vi "Read All Analog.vi"(0 "connection ID":refnum<k16>, 1 "address":u32, 2 "port":u16, 9 "timeout ms (1000)":i32=1000, 11 "error in (no error)":errorcluster) -> (4 "connection ID out":refnum<k16>, 6 "received data":string, 8 "Analog Values":u16[](array[numeric]), 15 "error out":errorcluster)   [LabVIEW 2016, in "instr.lvlib"]
doc: "Reads analog value all analog inputs and returns them as an array."
uses:
  instr.lvlib
panel:
  out "Send String":string
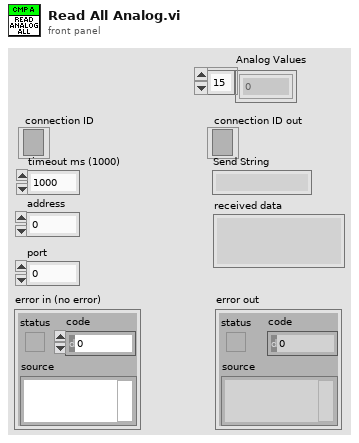
[diagram p1: front panel]
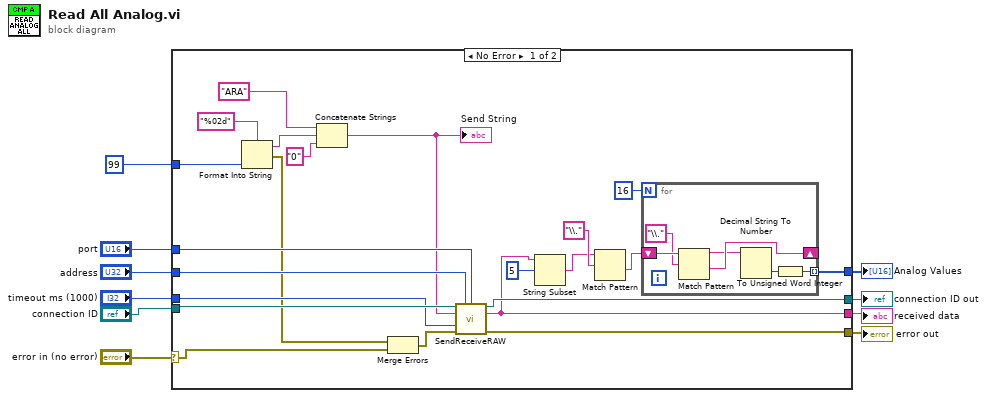
[diagram p0: block diagram]
diagram:
  n1 = case shown="No Error" "error in (no error)" {
    selector: "error in (no error)" -> [w22 w40]
    tunnel: [w32 w40] -> w10
    tunnel: "timeout ms (1000)" -> [w29 _]
    tunnel: "connection ID" -> [w30 w39]
    tunnel: [w31 w39] -> w6
    tunnel: "address" -> [w28 _]
    tunnel: "port" -> [w27 _]
    tunnel: [w12 _] -> w3
    tunnel: u16 99 ("Analog Number") -> [w23 _]
    tunnel: [w17 _] -> w1
    frame No Error {
      n2 = Format Into String(format string="%02d", w23) -> (resulting string=w24:string, error out=w19:errorcluster)  [unwired: 2 in]
      n3 = Concatenate Strings("ARA" ("data in"), w24, "0" ("string")) -> (w20:string)
      "Send String" <- w20
      n4 = Merge Errors(w19, w22) -> (w18:errorcluster)
      n5 = call "SendReceiveRAW.vi"("connection ID"=w30, "address"=w28, "port"=w27, "RAW data in"=w20, "timeout ms (1000)"=w29, "error in (no error)"=w18) -> ("connection ID out"=w31:refnum<k16>, "received data"=w12:string, "error out"=w32:errorcluster)  [unwired: 7 in]
      n6 = String Subset(string=w12, offset (0)=5 ("offset")) -> (substring=w11:string)  [unwired: 1 in]
      n7 = Match Pattern(string=w11, regular expression="\\.") -> (after substring=w15:string)  [unwired: 1 in, 3 out]
      n8 = for {
        N: 16 -> [_]
        tunnel: [w37] -> w17 mode=indexing
        shift-right: [w34] -> _
        shift-left: w15 -> [w36]
        n9 = Match Pattern(string=w36, regular expression="\\.") -> (before substring=w33:string, after substring=w34:string)  [unwired: 1 in, 2 out]
        n10 = Decimal String To Number(string=w33) -> (number=w38:i32)  [unwired: 2 in, 1 out]
        n11 = To Unsigned Word Integer(number=w38) -> (unsigned 16bit integer=w37:u16)
      }
    }
    frame Error {
    }
  }
  "error out" <- w10
  "received data" <- w3
  "connection ID out" <- w6
  "Analog Values" <- w1
